vi "Queue Is Nested.vi"(10 "Alias":string, 11 "jettl Event Actor in":refnum<class "jettl Event Actor.lvclass">) -> (2 "Queue Is Nested?":bool)   [LabVIEW 2021, in "jettl Event Actor.lvlib" / "jettl Event Actor.lvclass"]
uses:
  jettl Event Actor.lvclass
  jettl Event Actor.lvclass/jettl Event Actor.ctl
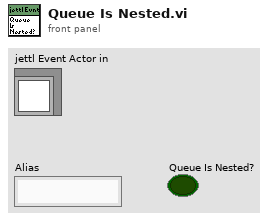
[diagram p1: front panel]
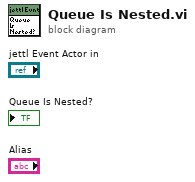
[diagram p0: block diagram]
diagram:
